vi "K Factor Loss.vi"(9 "K":dbl, 10 "Density (kg/m^3)":dbl, 11 "Velocity (m/s)":dbl) -> (3 "Loss (Pa)":dbl)   [LabVIEW 2019]
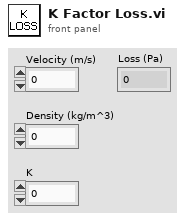
[diagram p1: front panel]
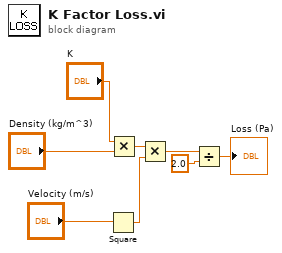
[diagram p0: block diagram]
diagram:
  n1 = Square(x="Velocity (m/s)") -> (x^2=w4:dbl)
  n2 = Multiply(x="K", y="Density (kg/m^3)") -> (x*y=w5:dbl)
  n3 = Multiply(x=w5, y=w4) -> (x*y=w6:dbl)
  n4 = Divide(x=w6, y=2.0) -> (x/y=→"Loss (Pa)":dbl)
